vi "Read PSU End of Charge.vi"(4 "error in":errorcluster) -> (0 "error out":errorcluster, 2 "End of Charge":bool)   [LabVIEW 2015]
uses:
  <vilib>/DAQmx/read.llb/DAQmx Read (Digital Bool 1Line 1Point).vi
  <vilib>/DAQmx/write.llb/DAQmx Write (Digital Bool 1Line 1Point).vi
  <vilib>/DAQmx/miscellaneous.llb/DAQmx Fill In Error Info.vi
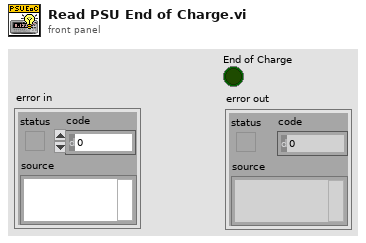
[diagram p1: front panel]
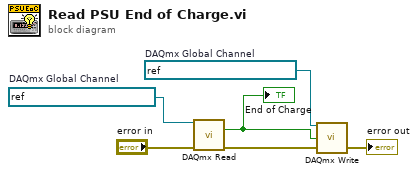
[diagram p0: block diagram]
diagram:
  w1 = refnum<k21> "DO9 End of Charge LED"  # DAQmx Global Channel
  w6 = refnum<k21> "DI0 PSU End of Charge"  # DAQmx Global Channel
  n1 = call-poly <vilib>:"DAQmx Read.vi"("task/channels in"=w6, "error in"="error in") -> ("data"=w2:bool, "error out"=w4:errorcluster)  [unwired: 11 in, 1 out]
  "End of Charge" <- w2
  n2 = call-poly <vilib>:"DAQmx Write.vi"("task/channels in"=w1, "data"=w2, "error in"=w4) -> ("error out"=→"error out":errorcluster)  [unwired: 10 in, 2 out]
